vi "make_axes_ticks_single_tick_line.vi"(0 "minor ticks":i32, 1 "major ticks":i32, 2 "Draw Major":bool, 3 "Draw Minor":bool, 4 "length":sgl, 5 "Color":u32(colorbox)) -> (14 "New Mesh Refnum":refnum<vi>)   [LabVIEW 2020, in "3DPC_SurfacePlot.xctl"]
uses:
  <vilib>/Native 3D Graph/xcontrol/3DPC_SurfacePlot.xctl
  <vilib>/picture/3D Picture Control/NI_3D Picture Control.lvlib
panel:
  in  "Use Display List?":bool=TRUE
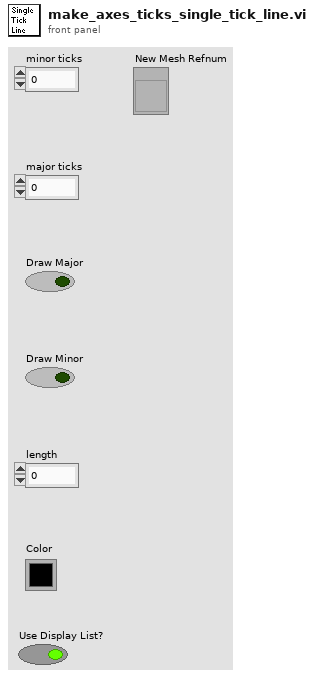
[diagram p1: front panel]
types:
  T1 = enum16{"Overall", "Per Primitive", "Per Vertex", "Binding Off"}
  T2 = enum16{"Points", "Lines", "Line Strip", "Line Loop", "Triangles", "Triangle Strip", "Triangle Fan", "Quads", "Quad Strip", "Polygon"}
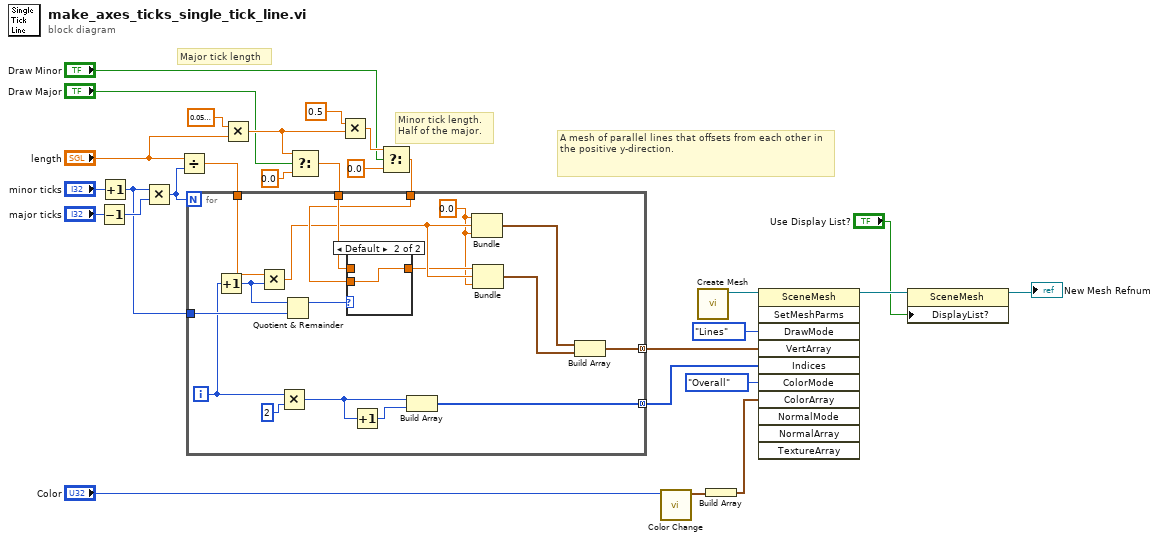
[diagram p0: block diagram]
diagram:
  # "A mesh of parallel lines that offsets from each other in the positive y-direction."
  # "Minor tick length.\nHalf of the major."
  # "Major tick length"
  n1 = Decrement(x="major ticks") -> (x-1=w15:i32)
  n2 = Increment(x="minor ticks") -> (x+1=w14:i32)
  n3 = Multiply(x=w14, y=w15) -> (x*y=w26:i32)
  n4 = Divide(x="length", y=w26) -> (x/y=w27:sgl)
  n5 = Multiply(x=sgl 0.05, y="length") -> (x*y=w10:sgl)
  n6 = Select(t=w10, s="Draw Major", f=sgl 0.0) -> (s? t:f=w3:sgl)
  n7 = Multiply(x=0.5, y=w10) -> (x*y=w7:dbl)
  n8 = Select(t=w7, s="Draw Minor", f=sgl 0.0) -> (s? t:f=w8:dbl)
  n9 = for {
    N: w26 -> [_]
    tunnel: w27 -> [w45]
    tunnel: w14 -> [w44]
    tunnel: w3 -> [w43]
    tunnel: w8 -> [w42]
    tunnel: [w31] -> w2 mode=concatenating
    tunnel: [w30] -> w1 mode=concatenating
    i -> [w33]
    w29 = 0.0
    n10 = Increment(x=w33) -> (x+1=w32:i32)
    n11 = Multiply(x=w45, y=w32) -> (x*y=w40:sgl)
    n12 = Multiply(x=w33, y=2) -> (x*y=w34:i32)
    n13 = Quotient & Remainder(x=w32, y=w44) -> (x-y*floor(x/y)=w41:i32)  [unwired: 1 out]
    n14 = case shown="Default" w41 {
      tunnel: w43 -> [w46 _]
      tunnel: w42 -> [_ w47]
      tunnel: [w46 w47] -> w39
      frame 0 {
      }
      frame Default {
      }
    }
    n15 = Increment(x=w34) -> (x+1=w35:i32)
    n16 = Build Array(w34, w35) -> (w30:i32[])
    n17 = Bundle(w29, w40, w29) -> (w38:cluster{dbl, sgl, dbl})  [unwired: 1 out]
    n18 = Bundle("f"=w39, w40, w29) -> (w37:cluster{"f":dbl, sgl, dbl})  [unwired: 1 out]
    n19 = Build Array(w38, w37) -> (w31:cluster{"f":dbl, sgl, dbl}[])
  }
  n20 = call <vilib>:"Color Change.vi"("Color"="Color") -> ("RGBA"=w17:cluster{"R":sgl, "G":sgl, "B":sgl, "A":sgl})  [unwired: 1 in, 9 out]
  n21 = call <vilib>:"Create Mesh.vi"() -> ("New Mesh Refnum"=w21:refnum<vi>)  [unwired: 1 in, 10 out]
  n22 = Build Array(w17) -> (w16:cluster{"R":sgl, "G":sgl, "B":sgl, "A":sgl}[])
  n23 = invoke class="SceneMesh" method="SetMeshParms"(reference=w21, "DrawMode"=T2."Lines" ("Draw Mode"), "VertArray"=w2, "Indices"=w1, "ColorMode"=T1."Overall" ("Color Binding Mode"), "ColorArray"=w16) -> (reference out=w13:refnum<vi>)  [unwired: 5 in, 10 out]
  n24 = property class="SceneMesh"(reference=w13, "DisplayList?"="Use Display List?") -> (reference out=→"New Mesh Refnum":refnum<vi>)  [unwired: 1 in, 1 out]
